vi "Read from Hardware.vi"(8 "error in":errorcluster, 10 "Values in":dbl[](array[numeric]), 11 "AIM ARINC-429 logging execution unit in":refnum<class "Logging Execution Unit.lvclass">) -> (0 "error out":errorcluster, 2 "Values out":dbl[](array[numeric]), 3 "AIM ARINC-429 logging execution unit out":refnum<class "Logging Execution Unit.lvclass">)   [LabVIEW 2020, in "AIM ARINC 429 Engine.lvlib" / "Implementation.lvlib" / "Logging Execution Unit.lvclass"]
uses:
  Logging Execution Unit.lvclass
  Execution Unit/Execution Unit.lvclass
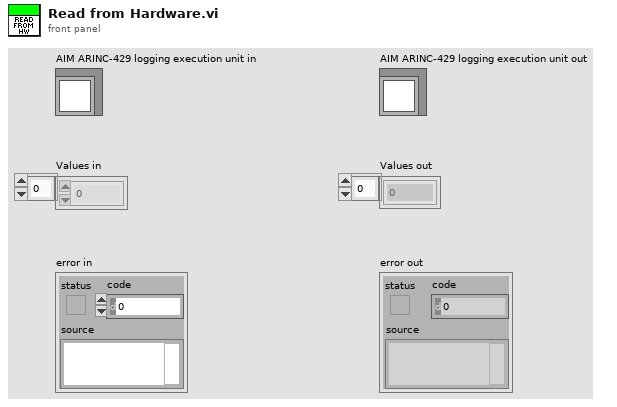
[diagram p1: front panel]
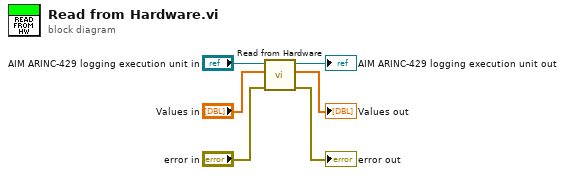
[diagram p0: block diagram]
diagram:
  n1 = call-parent "Read from Hardware.vi"("error in"="error in", "Values in"="Values in", "Ballard ARINC-429 Execution Unit in"="AIM ARINC-429 logging execution unit in") -> ("error out"=→"error out":errorcluster, "Values out"=→"Values out":dbl[], "Ballard ARINC-429 Execution Unit out"=→"AIM ARINC-429 logging execution unit out":refnum<class "Logging Execution Unit.lvclass">)  [unwired: 6 in]
